vi "Set Encoder Settings.vi"(8 "error in (no error)":errorcluster, 10 "Encoder Settings":T1 {"Encoder Filter" max=255; "Backlash Period (s)" min=0.0005 max=10.0 step=0.0005; "Multiplier" min=1 max=100000; "Counts/mm" min=1 max=100000}, 11 "Axis No.":u8) -> (0 "error out":errorcluster)   [LabVIEW 2026, in "MicroPulse_Driver.lvlib"]
uses:
  MicroPulse_Driver.lvlib
  Data/Datatypes/MP - encoder settings.ctl
  Data/Datatypes/MP - encoder type.ctl
  <instrlib>/Micropulse/Micropulse.lvlib
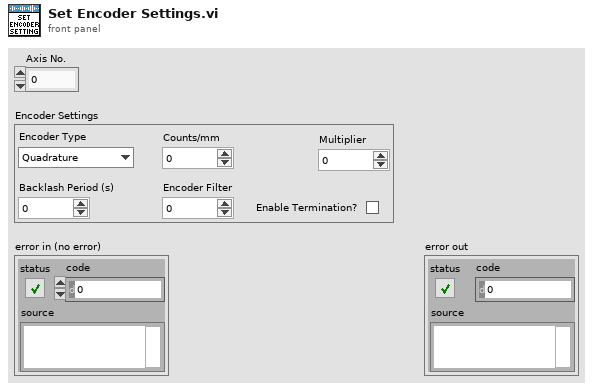
[diagram p1: front panel]
types:
  T1 = typedef "Micropulse.lvlib/MP - encoder settings.ctl" = cluster{"Encoder Type":T2, "Counts/mm":u32, "Enable Termination?":bool, "Multiplier":u32, "Backlash Period (s)":dbl, "Encoder Filter":u32}
  T2 = typedef "Micropulse.lvlib/MP - encoder type.ctl" = enum16{"Quadrature", "Step/Direction"}
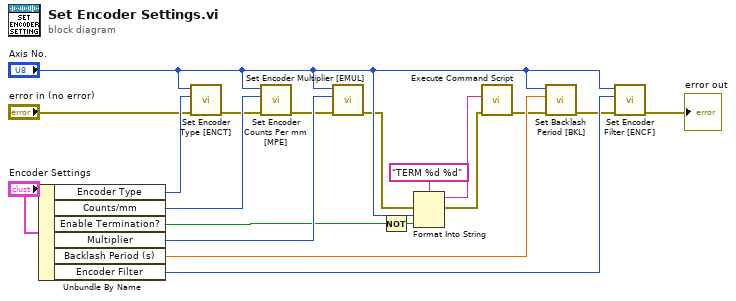
[diagram p0: block diagram]
diagram:
  n1 = Unbundle By Name("Encoder Settings") -> ("Encoder Type"=w11:T2, "Counts/mm"=w13:u32, "Enable Termination?"=w5:bool, "Multiplier"=w15:u32, "Backlash Period (s)"=w16:dbl, "Encoder Filter"=w18:u32)
  n2 = call "Set Encoder Type [ENCT].vi"("error in (no error)"="error in (no error)", "Encoder Type"=w11, "Axis No."="Axis No.") -> ("error out"=w12:errorcluster)  [unwired: 7 in, 1 out]
  n3 = call "Set Encoder Counts Per mm [MPE].vi"("error in (no error)"=w12, "Counts Per mm"=w13, "Axis No."="Axis No.") -> ("error out"=w14:errorcluster)  [unwired: 7 in, 1 out]
  n4 = call "Set Encoder Multiplier [EMUL].vi"("error in (no error)"=w14, "Multiplier"=w15, "Axis No."="Axis No.") -> ("error out"=w2:errorcluster)  [unwired: 7 in, 1 out]
  n5 = Not(x=w5) -> (.not. x?=w6:bool)
  n6 = Format Into String(format string="TERM %d %d", error in=w2, "Axis No.", w6) -> (resulting string=w3:string, error out=w1:errorcluster)  [unwired: 1 in]
  n7 = call "Execute Command Script.vi"("error in (no error)"=w1, "String in"=w3) -> ("error out"=w8:errorcluster)  [unwired: 7 in, 2 out]
  n8 = call "Set Backlash Period [BKL].vi"("error in (no error)"=w8, "Backlash Period (s)"=w16, "Axis No."="Axis No.") -> ("error out"=w17:errorcluster)  [unwired: 7 in, 1 out]
  n9 = call "Set Encoder Filter [ENCF].vi"("error in (no error)"=w17, "Filter"=w18, "Axis No."="Axis No.") -> ("error out"=→"error out":errorcluster)  [unwired: 7 in, 1 out]
